vi "TestSimpleNetOConvert.vi"() -> ()   [LabVIEW 2017]
panel:
  out ".NET object":refnum<k24>
  in  "Array":dbl[](array[numeric])
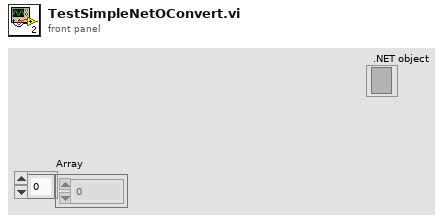
[diagram p1: front panel]
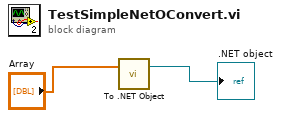
[diagram p0: block diagram]
diagram:
  n1 = call <vilib>:"To .NET Object.vi"("anything"="Array") -> (".NET object"=→".NET object":refnum<k24>)  [unwired: 1 in, 1 out]
